vi "LVITX Generate Folder Index.vi"(10 "File or Folder Path":path, 11 "All Files in Dir":path[](array[path])) -> ()   [LabVIEW 2013]
uses:
  <vilib>/Utility/file.llb/Write To Spreadsheet File (string).vi
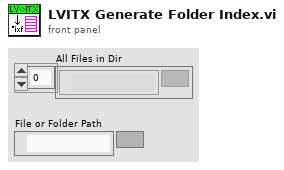
[diagram p1: front panel]
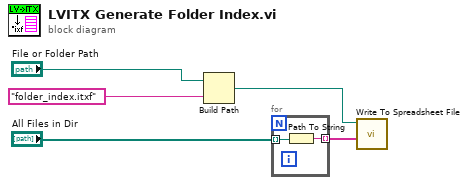
[diagram p0: block diagram]
diagram:
  n1 = Build Path(base path="File or Folder Path", name or relative path="folder_index.itxf") -> (appended path=w1:path)
  n2 = for {
    tunnel: "All Files in Dir" -> [w6] mode=indexing
    tunnel: [w7] -> w4 mode=indexing
    n3 = Path To String(path=w6) -> (string=w7:string)
  }
  n4 = call-poly <vilib>:"Write To Spreadsheet File.vi"("1D data"=w4, "file path (dialog if empty)"=w1) -> ()  [unwired: 6 in, 1 out]
